vi "GetUTCOffset.vi"(1 "Time":timestamp) -> (0 "UTC Offset (In Seconds)":u32)   [LabVIEW 2013]
panel:
  in  "7/1/2000 (Local)":T1
  in  "1/1/2000 (Local)":T1
  # "Return the Offset from GMT for the given Time\n(Given time is displayed in local time)"
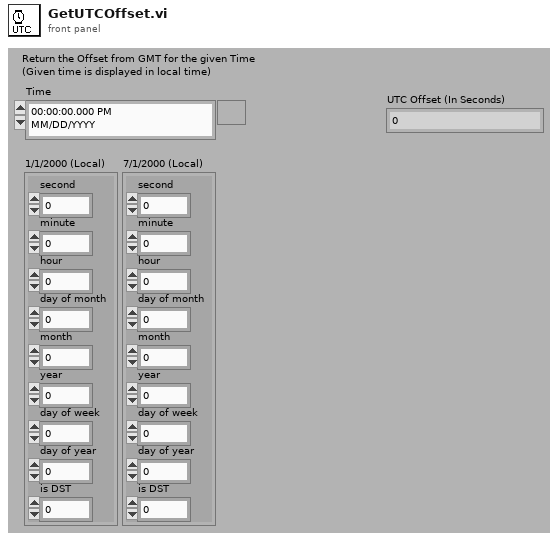
[diagram p1: front panel]
types:
  T1 = cluster{"second":i32, "minute":i32, "hour":i32, "day of month":i32, "month":i32, "year":i32, "day of week":i32, "day of year":i32, "is DST":i32}
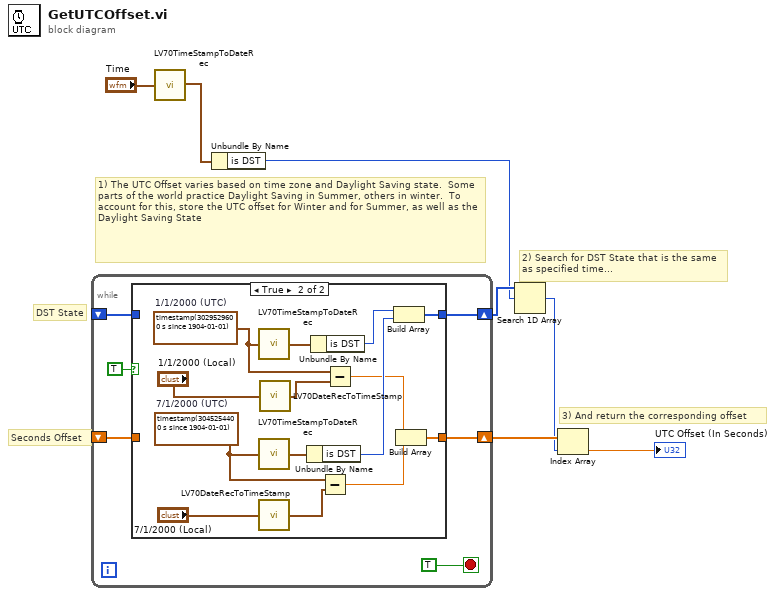
[diagram p0: block diagram]
diagram:
  # "3) And return the corresponding offset"
  # "2) Search for DST State that is the same\nas specified time..."
  # "Seconds Offset"
  # "DST State"
  # "1) The UTC Offset varies based on time zone and Daylight Saving state.  Some parts of the world practice Daylight Saving in Summer, others in winter.  To account for this, store the UTC offset for Winter and for Summer, as well as the Daylight Saving State"
  n1 = while {
    shift-right: [w11] -> w5
    shift-left: _ -> [w10]
    shift-right: [w12] -> w3
    shift-left: _ -> [w9]
    stop <- TRUE stop-if-true
    n2 = case shown="True" TRUE {
      tunnel: [w14 w25] -> w12
      tunnel: [w15 w24] -> w11
      tunnel: w10 -> [w15 _]
      tunnel: w9 -> [w14 _]
      frame False {
      }
      frame True {
        w19 = timestamp(3045254400 s since 1904-01-01)  # 7/1/2000 (UTC)
        w21 = timestamp(3029529600 s since 1904-01-01)  # 1/1/2000 (UTC)
        n3 = call <vilib>:"LV70TimeStampToDateRec.vi"("time stamp"=w21) -> ("date time rec"=w29:T1)
        n4 = call <vilib>:"LV70TimeStampToDateRec.vi"("time stamp"=w19) -> ("date time rec"=w28:T1)
        n5 = call <vilib>:"LV70DateRecToTimeStamp.vi"("date time rec"="7/1/2000 (Local)") -> ("Time Stamp"=w18:timestamp)
        n6 = call <vilib>:"LV70DateRecToTimeStamp.vi"("date time rec"="1/1/2000 (Local)") -> ("Time Stamp"=w20:timestamp)
        n7 = Unbundle By Name(w28) -> ("is DST"=w26:i32)
        n8 = Unbundle By Name(w29) -> ("is DST"=w27:i32)
        n9 = Subtract(x=w19, y=w18) -> (x-y=w16:dbl)
        n10 = Subtract(x=w21, y=w20) -> (x-y=w17:dbl)
        n11 = Build Array(w27, w26) -> (w24:i32[])
        n12 = Build Array(w17, w16) -> (w25:dbl[])
      }
    }
  }
  n13 = call <vilib>:"LV70TimeStampToDateRec.vi"("time stamp"="Time") -> ("date time rec"=w6:T1)
  n14 = Unbundle By Name(w6) -> ("is DST"=w4:i32)
  n15 = Search 1D Array(1D array=w5, element=w4) -> (index of element=w1:i32)  [unwired: 1 in]
  n16 = Index Array(array=w3, index=w1) -> (element=→"UTC Offset (In Seconds)":dbl)
